vi "Close Tuner.vi"(8 "error in (no error)":errorcluster, 11 "iTuner reference in":refnum<k7>) -> (0 "error out":errorcluster)   [LabVIEW 2016, in "FocusTuner.lvlib"]
doc: "Re-initializes all axes of the tuner to its home position before terminating the software connection to the instrument."
uses:
  FocusTuner.lvlib
  <instrlib>/Focus iTuner Series/Public/Action-Status/Initialize Tuner (All Axes).vi
  <instrlib>/Focus iTuner Series/Focus iTuner Series.lvlib
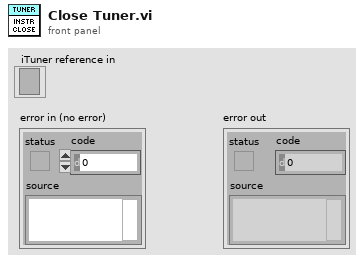
[diagram p1: front panel]
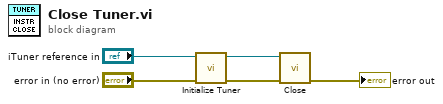
[diagram p0: block diagram]
diagram:
  n1 = call-poly <instrlib>:"Initialize Tuner.vi"("error in (no error)"="error in (no error)", "iTuner reference in"="iTuner reference in") -> ("error out"=w4:errorcluster, "iTuner reference out"=w5:refnum<k7>)  [unwired: 8 in]
  n2 = call <instrlib>:"Close.vi"("error in (no error)"=w4, "iTuner reference in"=w5) -> ("error out"=→"error out":errorcluster)  [unwired: 9 in]
